vi "tm_opendcimgfile.vi"(8 "error in (no error)":errorcluster, 11 "Path":path) -> (0 "error out":errorcluster, 2 "Total Frames":i32, 3 "File Handle":u32)   [LabVIEW 2015]
uses:
  tmcamcon.dll
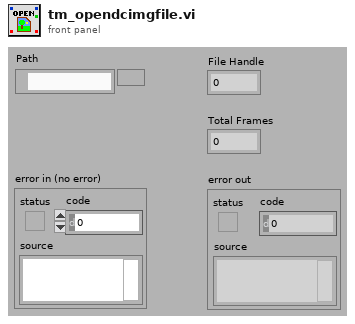
[diagram p1: front panel]
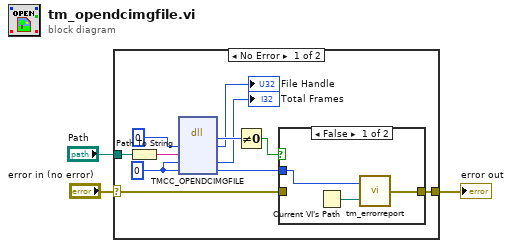
[diagram p0: block diagram]
diagram:
  n1 = case shown="No Error" "error in (no error)" {
    selector: "error in (no error)" -> [w8 w19]
    tunnel: [w5 w19] -> w2
    tunnel: "Path" -> [w10 _]
    frame No Error {
      w4 = 0 ("totalframes")
      n2 = Path To String(path=w10) -> (string=w9:string)
      n3 = dll-call lib="tmcamcon.dll" fn="TMCC_OPENDCIMGFILE"("filehandle"=u32 0, "path"=w9, "totalframes"=w4, "Erval"=w4) -> ("return type"=w14:u32, "filehandle"=→"File Handle":u32, "totalframes"=→"Total Frames":i32, "Erval"=w7:i32)  [unwired: 4 in, 2 out]
      n4 = Not Equal To 0?(x=w14) -> (x != 0?=w6:bool)
      n5 = case shown="False" w6 {
        tunnel: w8 -> [_ w18]
        tunnel: [w16 w18] -> w5
        tunnel: w7 -> [w15 _]
        frame False {
          n6 = Current VI's Path() -> (path=w17:path)
          n7 = call "tm_errorreport.vi"("Source"=w17, "Error"=w15) -> ("error out"=w16:errorcluster)
        }
        frame True {
        }
      }
    }
    frame Error {
    }
  }
  "error out" <- w2
